vi "sam_mlotek_z_pxi.vi"() -> ()   [LabVIEW 2020]
doc: "This example demonstrates how to continuously acquire buffered acceleration, sound pressure, or force measurements from IEPE sensors using a DAQmx device.\n\nFor instructions on how to connect your signals to the DAQ device, refer to your device documentation."
uses:
  <vilib>/Utility/error.llb/DialogType.ctl
  <vilib>/DAQmx/read.llb/DAQmx Read (Analog 1D Wfm NChan NSamp).vi
  <vilib>/DAQmx/create/channels.llb/DAQmx Create Channel (AI-Force-IEPE Sensor).vi
  <vilib>/DAQmx/configure/timing.llb/DAQmx Timing (Sample Clock).vi
  <vilib>/DAQmx/miscellaneous.llb/DAQmx Fill In Error Info.vi
  <vilib>/measure/mascope.llb/Amplitude and Levels N chan.vi
  <vilib>/Utility/file.llb/Write Delimited Spreadsheet (DBL).vi
  <resource>/objmgr/daqmx.rc
  <vilib>/measure/NI_MAPro.lvlib
panel:
  out "Analog Data 2":dynamicdata(graph)
  in  "file (use dialog)":path
  out "amplitude 2":dbl format="%.1f"
  out "amplitude 1":dbl format="%.1f"
  out "Analog Data":waveform(dbl)[](graph)
  in  "Sensitivity":dbl=10.2
  in  "Min Force":dbl=-300.0
  in  "Max Force":dbl=300.0
  in  "Sensitivity Units":i32(ring)=15892 items=["mVolts/N"=15891, "mVolts/lb"=15892]
  in  "Force Units":i32(ring)=15875 items=["Newtons"=15875, "Pounds"=15876, "From Custom Scale"=10065]
  out "F max [N]":dbl format="%.1f"
  in  "IEPE Current Value (A)":dbl=0.004
  in  "IEPE Excitation Source":i32(ring)=10200 items=["Internal"=10200, "External"=10167, "None"=10230]
  in  "Terminal Configuration":i32(ring)=-1 items=["default"=-1, "RSE"=10083, "NRSE"=10078, "Differential"=10106, "Pseudodifferential"=12529]
  in  "Physical Channel":tag="cDAQ2Mod1/ai0"
  in  "Stop":bool
  out "Waveform Graph":waveform(dbl)[](graph)
  in  "Samples per Loop":i32=100
  in  "Sample Rate":dbl=1000.0
  in  "Sample Clock Source":tag="OnboardClock"
  out "Actual Sample Rate":dbl=1000.0000111176631 format="%0.2f"
  # "Channel Settings"
  # "Acquired Data"
  # "Scope Settings"
  # "Timing Settings"
  # "Logging Settings"
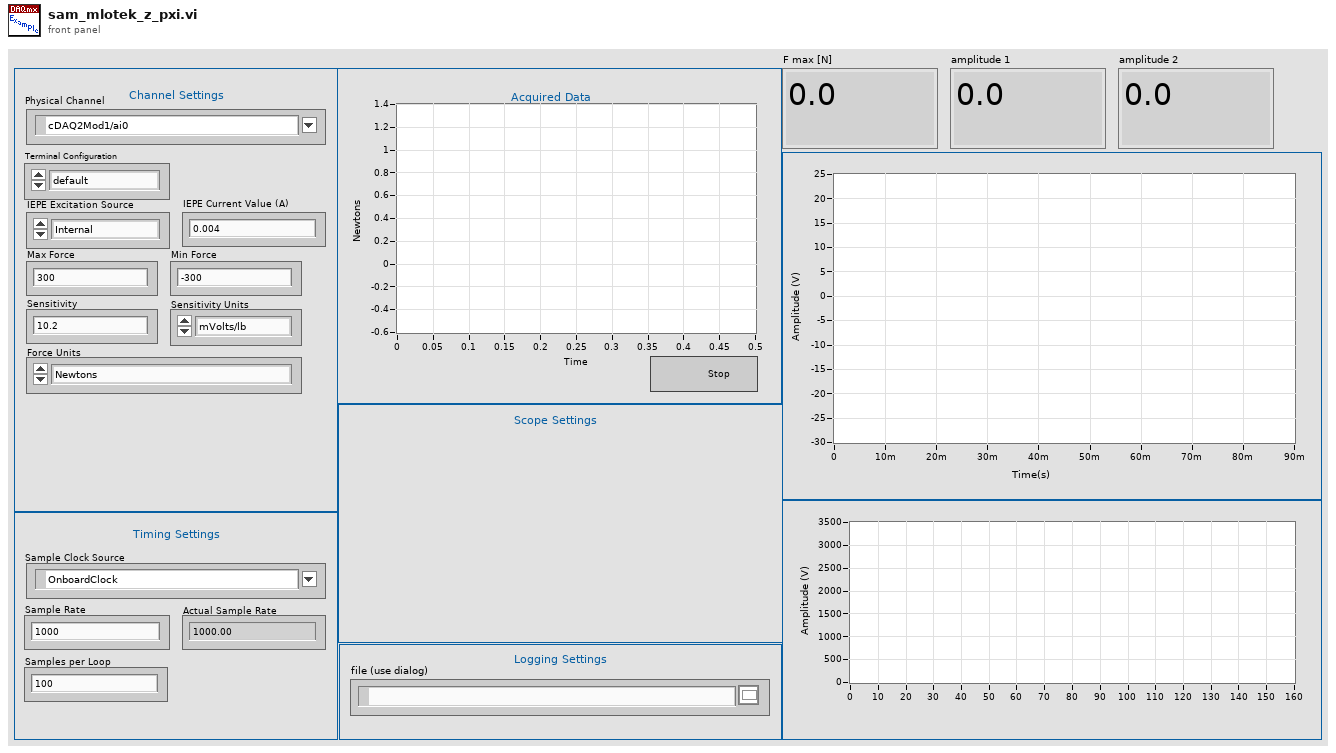
[diagram p1: front panel]
types:
  T1 = typedef "DialogType.ctl" = u16
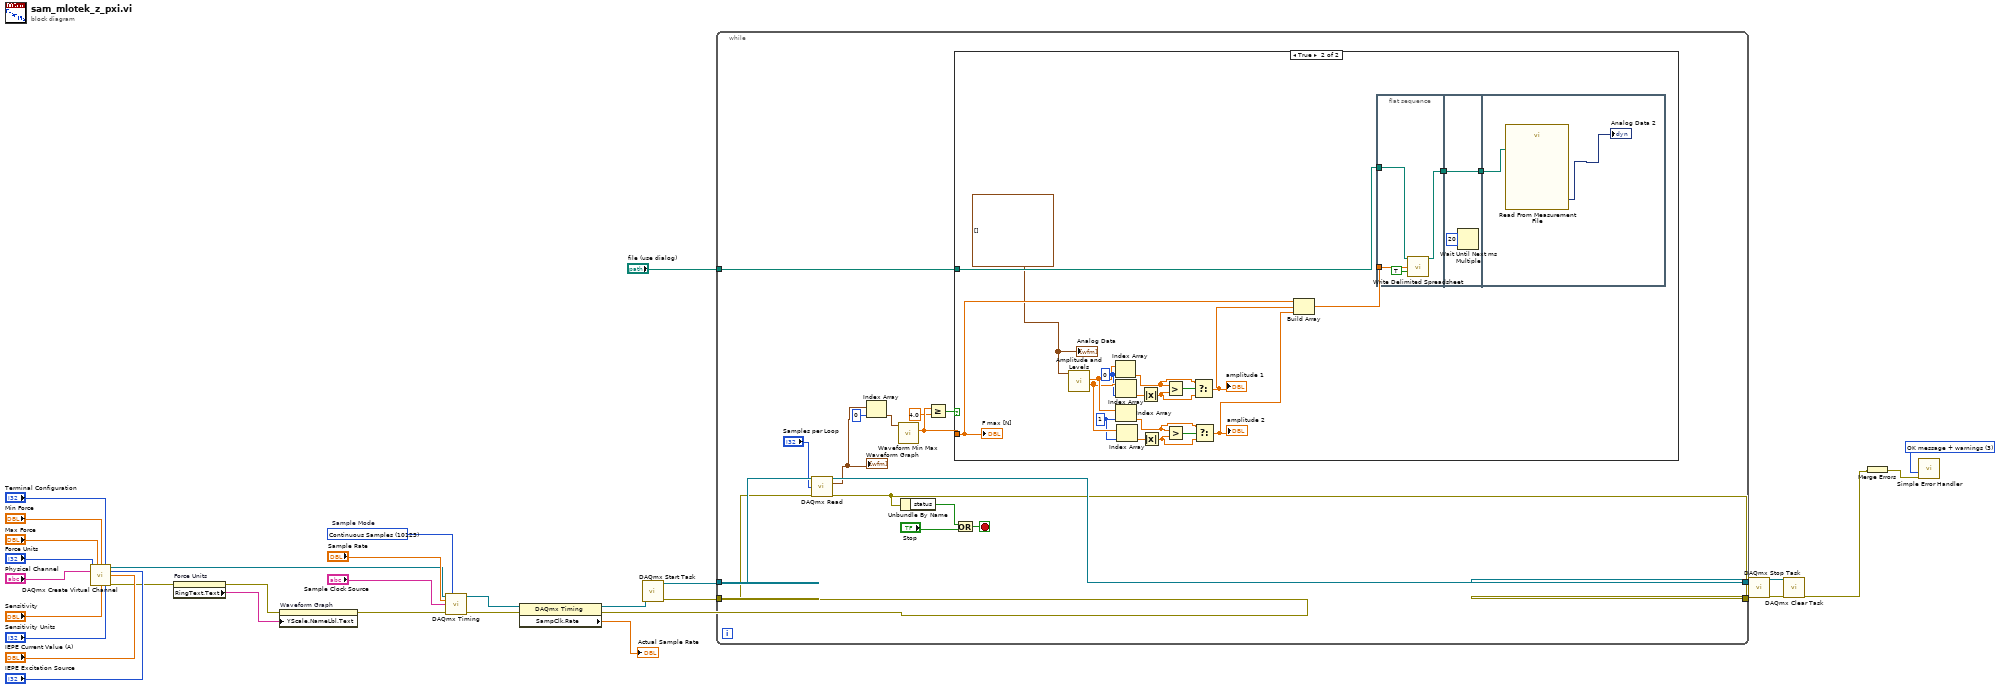
[diagram p0: block diagram]
diagram:
  w15 = T1 3 items=["no dialog", "OK message", "continue or stop message", "OK message + warnings", "continue/stop + warnings"] ("type of dialog (OK msg:1)")
  w30 = 10123 items=["Finite Samples"=10178, "Continuous Samples"=10123, "Hardware Timed Single Point"=12522]  # Sample Mode
  n1 = call-poly <vilib>:"DAQmx Create Virtual Channel.vi"("maximum value"="Max Force", "minimum value"="Min Force", "input terminal configuration"="Terminal Configuration", "physical channels"="Physical Channel", "current excitation source"="IEPE Excitation Source", "current excitation value"="IEPE Current Value (A)", "units"="Force Units", "sensitivity"="Sensitivity", "sensitivity units"="Sensitivity Units") -> ("task out"=w4:refnum<k21>, "error out"=w12:errorcluster)  [unwired: 5 in]
  n2 = property on="Force Units" class="Ring (strict)"(error in=w12) -> (error out=w6:errorcluster, "RingText.Text"=w5:string)  [unwired: 1 in, 1 out]
  n3 = property on="Waveform Graph" class="WFGraph (strict)"(error in=w6, "YScale.NameLbl.Text"=w5) -> (error out=w20:errorcluster)  [unwired: 1 in, 1 out]
  n4 = call-poly <vilib>:"DAQmx Timing.vi"("task/channels in"=w4, "sample mode"=w30, "rate"="Sample Rate", "source"="Sample Clock Source", "error in"=w20) -> ("task out"=w32:refnum<k21>, "error out"=w31:errorcluster)  [unwired: 9 in]
  n5 = property class="DAQmx Timing"(reference=w32, error in=w31) -> (reference out=w13:refnum<k21>, error out=w14:errorcluster, "SampClk.Rate"=→"Actual Sample Rate":dbl)
  n6 = call <vilib>:"DAQmx Start Task.vi"("task/channels in"=w13, "error in"=w14) -> ("task out"=w29:refnum<k21>, "error out"=w28:errorcluster)  [unwired: 12 in]
  n7 = while {
    tunnel: w29 -> [w47]
    tunnel: w28 -> [w46]
    tunnel: [w43] -> w16
    tunnel: [w44] -> w17
    tunnel: "file (use dialog)" -> [w33]
    stop <- w45 stop-if-true
    n8 = call-poly <vilib>:"DAQmx Read.vi"("task/channels in"=w47, "number of samples per channel"="Samples per Loop", "error in"=w46) -> ("task out"=w44:refnum<k21>, "data"=w39:waveform(dbl)[], "error out"=w43:errorcluster)  [unwired: 10 in]
    "Waveform Graph" <- w39
    n9 = Index Array(array=w39, index=0) -> (element=w37:waveform(dbl))
    n10 = call <vilib>:"Waveform Min Max.vi"("waveform in"=w37) -> ("Y max"=w36:dbl)  [unwired: 5 in, 5 out]
    n11 = Unbundle By Name(w43) -> ("status"=w42:bool)
    n12 = Greater Or Equal?(x=w36, y=4.0) -> (x >= y?=w34:bool)
    n13 = case shown="True" w34 {
      tunnel: w36 -> [_ w51]
      tunnel: w33 -> [_ w54]
      frame False {
      }
      frame True {
        w48 = waveform(dbl)[] [] ("Analog Data")
        w56 = 1 ("index")
        w57 = 0 ("index")
        n14 = call-poly <vilib>:"Amplitude and Levels.vi"("signal(s) in"=w48) -> ("low state level"=w58:dbl[], "high state level"=w59:dbl[])  [unwired: 7 in, 2 out]
        n15 = Index Array(array=w59, index=w57) -> (element=w64:dbl)
        n16 = Index Array(array=w58, index=w57) -> (element=w65:dbl)
        n17 = Index Array(array=w59, index=w56) -> (element=w63:dbl)
        n18 = Index Array(array=w58, index=w56) -> (element=w62:dbl)
        n19 = Absolute Value(x=w65) -> (abs(x)=w67:dbl)
        n20 = Absolute Value(x=w62) -> (abs(x)=w60:dbl)
        n21 = Greater?(x=w64, y=w67) -> (0:w66:bool)
        n22 = Greater?(x=w63, y=w60) -> (0:w61:bool)
        n23 = Select(t=w64, s=w66, f=w67) -> (s? t:f=w52:dbl)
        "amplitude 1" <- w52
        n24 = Select(t=w63, s=w61, f=w60) -> (s? t:f=w55:dbl)
        "amplitude 2" <- w55
        n25 = Build Array(w51, w52, w55) -> (w53:dbl[])
        n26 = flat-sequence {
          tunnel: w54 -> [w69]
          tunnel: w53 -> [w71]
          tunnel: [w68] -> w50
          tunnel: w50 -> [w73]
          tunnel: [w73] -> w49
          tunnel: w49 -> [w75]
          frame #0 {
            n27 = call-poly <vilib>:"Write Delimited Spreadsheet.vi"("file path (dialog if empty)"=w69, "1D data"=w71, "append to file? (new file:F)"=TRUE) -> ("new file path (Not A Path if cancelled)"=w68:path)  [unwired: 11 in, 1 out]
          }
          frame #1 {
            n28 = Wait Until Next ms Multiple(millisecond multiple=u32 20) -> ()  [unwired: 1 out]
          }
          frame #2 {
            n29 = call "Read From Measurement File"("Filename"=w75) -> ("Signals"=→"Analog Data 2":dynamicdata)  [unwired: 5 in, 5 out]
          }
        }
        "F max [N]" <- w51
        "Analog Data" <- w48
      }
    }
    n30 = Or(x=w42, y="Stop") -> (x .or. y?=w45:bool)
  }
  n31 = call <vilib>:"DAQmx Stop Task.vi"("task/channels in"=w17, "error in"=w16) -> ("task out"=w19:refnum<k21>, "error out"=w18:errorcluster)  [unwired: 12 in]
  n32 = call <vilib>:"DAQmx Clear Task.vi"("task in"=w19, "error in"=w18) -> ("error out"=w3:errorcluster)  [unwired: 13 in]
  n33 = Merge Errors(w3) -> (w2:errorcluster)
  n34 = call <vilib>:"Simple Error Handler.vi"("type of dialog (OK msg:1)"=w15, "error in (no error)"=w2) -> ()  [unwired: 3 in, 5 out]
